vi "ToggleAllRooms.vi"(0 "object in":refnum<class "System.lvclass">, 5 "Error In":errorcluster) -> (14 "object out":refnum<class "System.lvclass">, 19 "Error Out":errorcluster)   [LabVIEW 2024, in "System.lvclass"]
doc: "Toggle all of the elements in all of the rooms"
uses:
  System.lvclass
panel:
  # "Connector Pane"
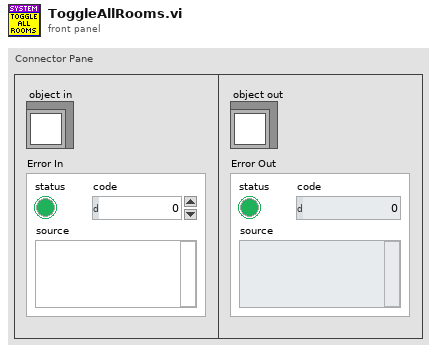
[diagram p1: front panel]
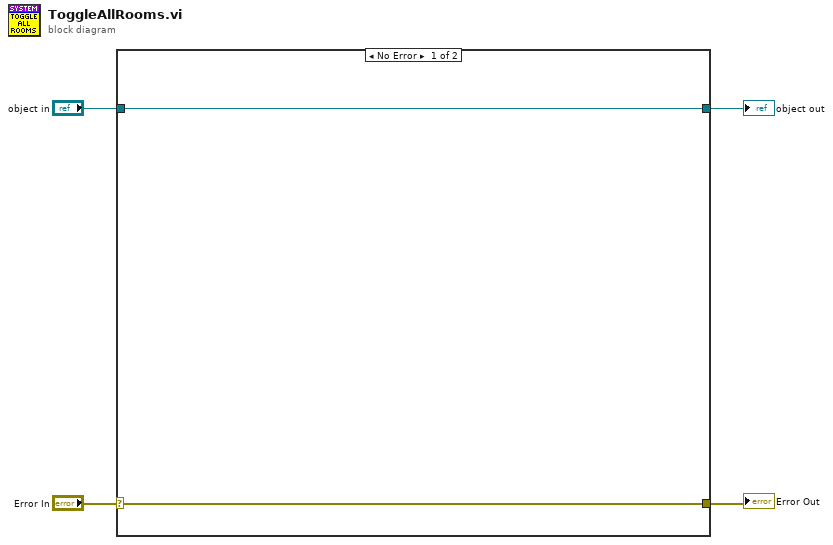
[diagram p0: block diagram]
diagram:
  n1 = case shown="No Error" "Error In" {
    selector: "Error In" -> [w5 w8]
    tunnel: [w5 w8] -> w3
    tunnel: [w6 w7] -> w1
    tunnel: "object in" -> [w6 w7]
    frame No Error {
    }
    frame Error {
    }
  }
  "Error Out" <- w3
  "object out" <- w1
